vi "Open TCP Connection.vi"(8 "error in (no error)":errorcluster, 9 "timeout ms (60000)":i32, 10 "remote port":u16, 11 "remote address":string) -> (0 "error out":errorcluster, 3 "TCP Connection out":refnum<class "TCP Connection.lvclass">)   [LabVIEW 2019, in "TCP Connection.lvclass"]
uses:
  TCP Connection.lvclass
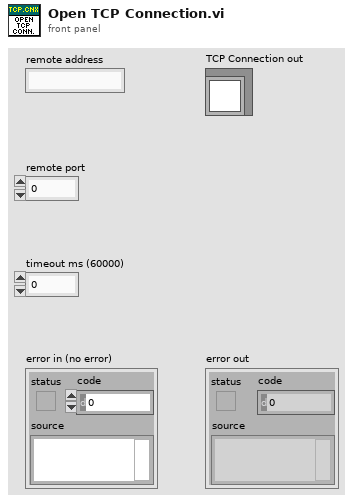
[diagram p1: front panel]
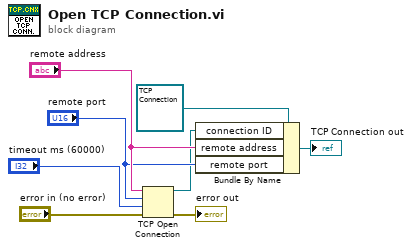
[diagram p0: block diagram]
diagram:
  n1 = TCP Open Connection(address="remote address", remote port or service name="remote port", timeout ms (60000)="timeout ms (60000)", error in (no error)="error in (no error)") -> (connection ID=w1:refnum<k5>, error out=→"error out":errorcluster)  [unwired: 1 in]
  n2 = Bundle By Name(cluster=refnum<class "TCP Connection.lvclass"> refnum ("TCP Connection out"), "connection ID"=w1, "remote address"="remote address", "remote port"="remote port") -> (→"TCP Connection out":refnum<class "TCP Connection.lvclass">)
